vi "CCD demand.vi"() -> ()   [LabVIEW 2017]
panel:
  in  "CCD demand":T1
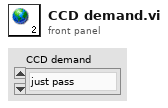
[diagram p1: front panel]
types:
  T1 = typedef "数据分析命令集.ctl" = enum16{"just pass", "calibration GPU", "calibration", "Z record", "tracking xy", "tracking XYZ", "tracking xy GPU", "tracking xyz GPU", "record xyz GPU"}
diagram:
